vi "1A Testbench for Steven's Defilter.vi"() -> ()   [LabVIEW 2011]
uses:
  <vilib>/ptbypt/NI_PtbyPt.lvlib
panel:
  in  "amplitude":dbl=1.0 format="%0.2f"
  in  "frequency":dbl=1.0 format="%0.2f"
  in  "phase":dbl format="%0.2f"
  in  "millisecond multiple":u32
  out "Waveform Chart":T1(graph)
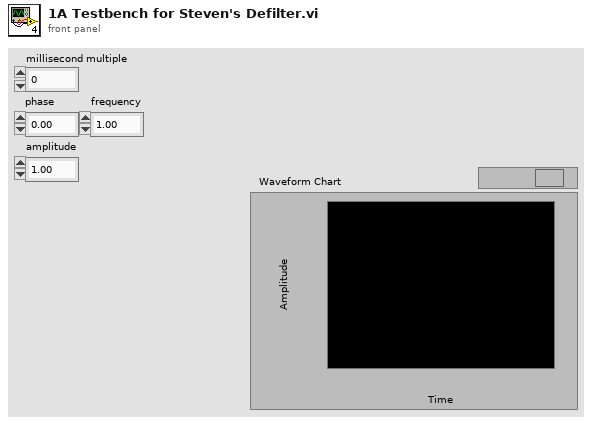
[diagram p1: front panel]
types:
  T1 = cluster{"sine wave":dbl, "Filtered Value Out":dbl}
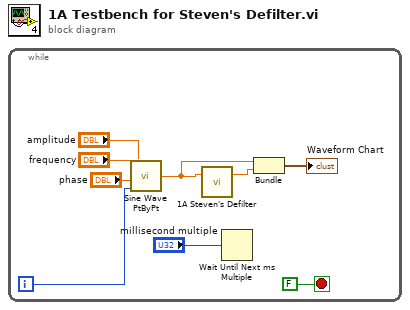
[diagram p0: block diagram]
diagram:
  n1 = while {
    i -> [w9]
    stop <- FALSE stop-if-true
    n2 = call <vilib>:"Sine Wave PtByPt.vi"("time"=w9, "phase"="phase", "frequency"="frequency", "amplitude"="amplitude") -> ("sine wave"=w6:dbl)
    n3 = call "1A Steven's Defilter.vi"("Value In"=w6) -> ("Filtered Value Out"=w7:dbl)  [unwired: 2 in]
    n4 = Wait Until Next ms Multiple(millisecond multiple="millisecond multiple") -> ()  [unwired: 1 out]
    n5 = Bundle("sine wave"=w6, "Filtered Value Out"=w7) -> (→"Waveform Chart":T1)  [unwired: 1 in]
  }
